vi "DrivePath-C.vi"(11 "Params":string[][](array[string])) -> ()   [LabVIEW 2017]
uses:
  RoutineData.vi
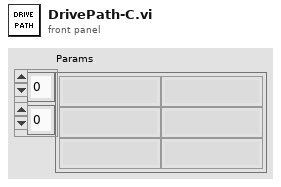
[diagram p1: front panel]
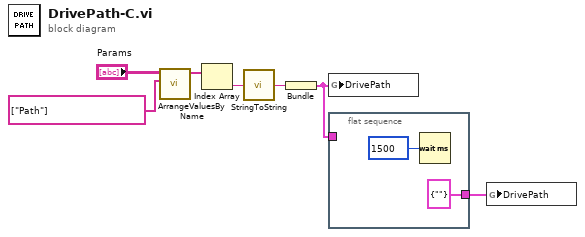
[diagram p0: block diagram]
diagram:
  n1 = call "ArrangeValuesByName.vi"("Names"=string[] ["Path"], "Names/Values in"="Params") -> ("Values Out"=w2:string[])  [unwired: 9 in]
  n2 = Index Array(array=w2) -> (element=w1:string)  [unwired: 1 in]
  n3 = call "StringToString.vi"("String"=w1) -> ("Output"=w6:string)
  n4 = Bundle("Output"=w6) -> (w7:cluster{"Output":string})  [unwired: 1 in]
  n5 = global write "RoutineData.vi" "DrivePath"(w7) -> ()
  n6 = flat-sequence {
    tunnel: w7 -> [_]
    tunnel: [cluster{"Path":string} {"Path"=""} ("DrivePath")] -> w5
    frame #0 {
      n7 = Wait (ms)(milliseconds to wait=u32 1500) -> ()  [unwired: 1 out]
    }
  }
  n8 = global write "RoutineData.vi" "DrivePath"(w5) -> ()
